vi "M02 Toy Factory.vi"(9 "Angle in":dbl format="%#_13g", 11 "EV3 in":T1) -> (3 "EV3 out":T1)   [LabVIEW 2016]
uses:
  <vilib>/NXT/Subs/LVHSConnector.ctl
  <vilib>/NXT/LegoClasses/BrickReference/BrickReference.lvclass
  <vilib>/NXT/Dual Mode Library/Waits/Wait_Num.vi
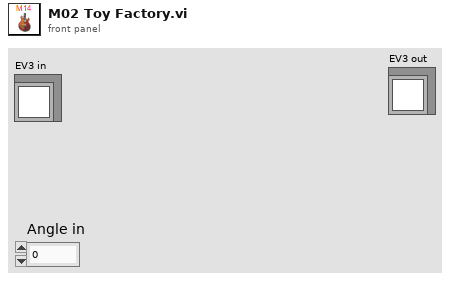
[diagram p1: front panel]
types:
  T1 = typedef "LVHSConnector.ctl" = refnum<class "BrickReference.lvclass">
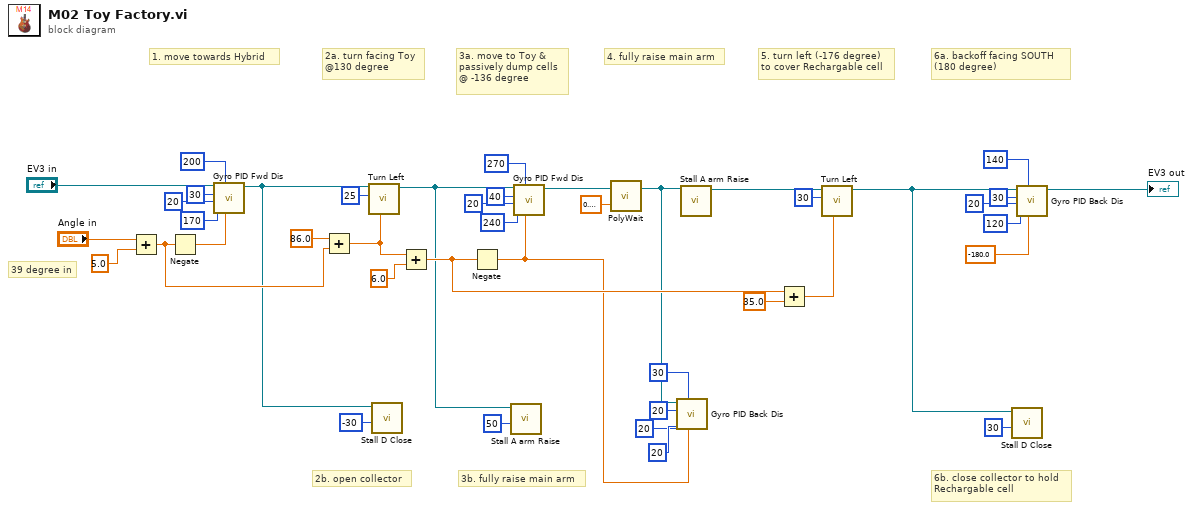
[diagram p0: block diagram]
diagram:
  # "3b. fully raise main arm"
  # "39 degree in"
  # "6b. close collector to hold\nRechargable cell"
  # "2b. open collector"
  # "6a. backoff facing SOUTH\n(180 degree)"
  # "5. turn left (-176 degree)\nto cover Rechargable cell"
  # "4. fully raise main arm"
  # "3a. move to Toy &\npassively dump cells\n@ -136 degree"
  # "2a. turn facing Toy\n@130 degree"
  # "1. move towards Hybrid"
  n1 = Add(x="Angle in", y=5.0) -> (x+y=w34:dbl)
  n2 = Negate(x=w34) -> (-x=w32:dbl)
  n3 = call "Gyro PID Fwd Dis.vi"("Target angle"=w32, "Threshold to stop"=200 ("Stop rotation"), "Threshold to slow"=170 ("Threshold to De-acc"), "Min. speed"=20 ("De-acc"), "Max. speed"=30 ("Acc"), "EV3 in"="EV3 in") -> ("EV3 out"=w14:T1)  [unwired: 5 in]
  n4 = Add(x=86.0, y=w34) -> (x+y=w40:dbl)
  n5 = call "Turn Left.vi"("Turning angle"=w40, "Motor B (right)"=i8 25, "EV3 in"=w14) -> ("EV3 out"=w10:T1)  [unwired: 8 in]
  n6 = call "Stall D Close.vi"("Power"=i8 -30, "NXT/EV3"=w14) -> ()  [unwired: 9 in, 1 out]
  n7 = Add(x=w40, y=6.0) -> (x+y=w20:dbl)
  n8 = Negate(x=w20) -> (-x=w1:dbl)
  n9 = call "Stall A arm Raise.vi"("Power"=i8 50, "NXT/EV3"=w10) -> ()  [unwired: 9 in, 1 out]
  n10 = call "Gyro PID Fwd Dis.vi"("Target angle"=w1, "Threshold to stop"=270 ("Stop rotation"), "Threshold to slow"=240 ("Threshold to De-acc"), "Min. speed"=20 ("De-acc"), "Max. speed"=40 ("Acc"), "EV3 in"=w10) -> ("EV3 out"=w27:T1)  [unwired: 5 in]
  n11 = call-poly <vilib>:"PolyWait.vi"("Time (1 sec)"=sgl 0.3, "NXT/EV3"=w27) -> ("NXT/EV3"=w6:T1)  [unwired: 2 in]
  n12 = call "Gyro PID Back Dis.vi"("Target angle"=w1, "Threshold to stop"=30, "Threshold to slow"=20, "Min. speed"=20, "Max. speed"=20, "EV3 in"=w6) -> ()  [unwired: 5 in, 1 out]
  n13 = call "Stall A arm Raise.vi"("NXT/EV3"=w6) -> ("NXT/EV3"=w26:T1)  [unwired: 10 in]
  n14 = Add(x=w20, y=35.0) -> (x+y=w15:dbl)
  n15 = call "Turn Left.vi"("Turning angle"=w15, "Motor B (right)"=i8 30, "EV3 in"=w26) -> ("EV3 out"=w8:T1)  [unwired: 8 in]
  n16 = call "Stall D Close.vi"("Power"=i8 30, "NXT/EV3"=w8) -> ()  [unwired: 9 in, 1 out]
  n17 = call "Gyro PID Back Dis.vi"("Target angle"=sgl -180.0, "Threshold to stop"=140, "Threshold to slow"=120, "Min. speed"=20, "Max. speed"=30, "EV3 in"=w8) -> ("EV3 out"=→"EV3 out":T1)  [unwired: 5 in]
